vi "Chirp_DFT_V3.vi"(8 "error in (no error)":errorcluster, 11 "ChirpV2 in":refnum<class "ChirpV2.lvclass">) -> (0 "error out":errorcluster, 3 "ChirpV2 out":refnum<class "ChirpV2.lvclass">)   [LabVIEW 2014, in "ChirpV2.lvclass"]
uses:
  ChirpV2.lvclass
  <vilib>/Analysis/2dsp.llb/Real FFT.vi
  <vilib>/Analysis/NI_AALPro.lvlib
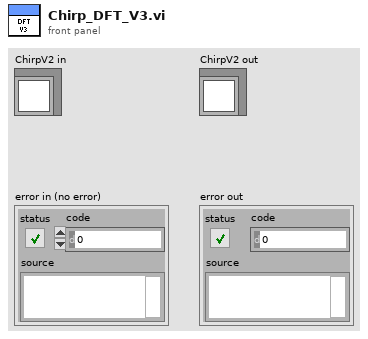
[diagram p1: front panel]
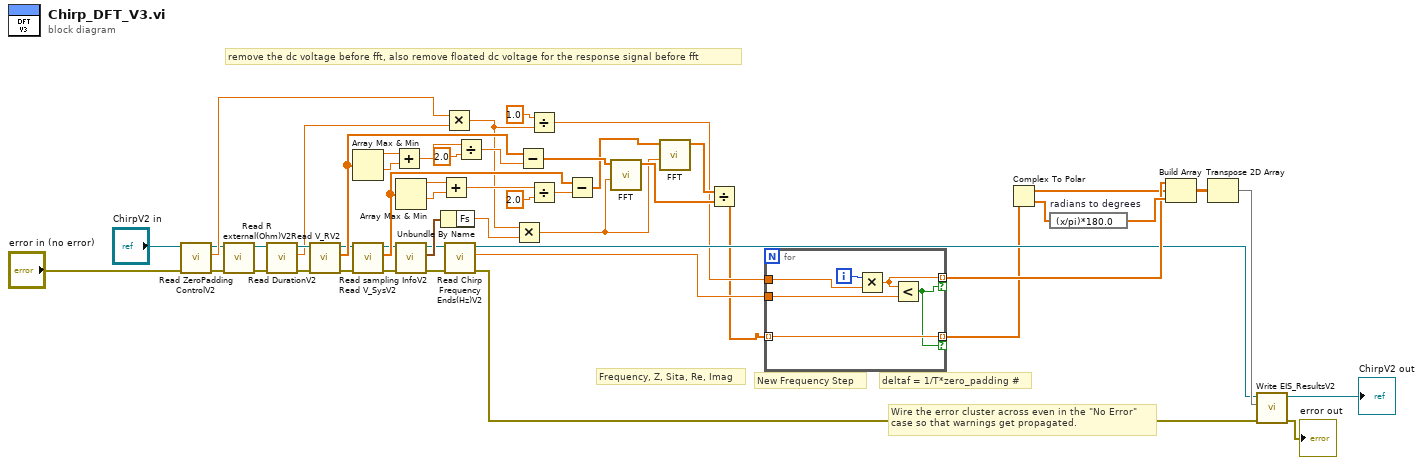
[diagram p0: block diagram]
diagram:
  # "deltaf = 1/T*zero_padding #"
  # "remove the dc voltage before fft, also remove floated dc voltage for the response signal before fft"
  # "Frequency, Z, Sita, Re, Imag"
  # "New Frequency Step"
  # "Wire the error cluster across even in the \"No Error\"\ncase so that warnings get propagated."
  n1 = call-dynamic "Read ZeroPadding ControlV2.vi"("error in (no error)"="error in (no error)", "ChirpV2 in"="ChirpV2 in") -> ("error out"=w49:errorcluster, "ZeroPadding Control"=w50:dbl, "ChirpV2 out"=w48:refnum<class "ChirpV2.lvclass">)  [unwired: 7 in]
  n2 = call-dynamic "Read R external(Ohm)V2.vi"("error in (no error)"=w49, "ChirpV2 in"=w48) -> ("error out"=w19:errorcluster, "ChirpV2 out"=w21:refnum<class "ChirpV2.lvclass">)  [unwired: 7 in, 1 out]
  n3 = call-dynamic "Read DurationV2.vi"("error in (no error)"=w19, "ChirpV2 in"=w21) -> ("error out"=w18:errorcluster, "Duration"=w17:dbl, "ChirpV2 out"=w20:refnum<class "ChirpV2.lvclass">)  [unwired: 7 in]
  n4 = call-dynamic "Read V_RV2.vi"("error in (no error)"=w18, "ChirpV2 in"=w20) -> ("error out"=w41:errorcluster, "V_R"=w42:dbl[], "ChirpV2 out"=w40:refnum<class "ChirpV2.lvclass">)  [unwired: 7 in]
  n5 = Array Max & Min(array=w42) -> (max value=w30:dbl, min value=w31:dbl)  [unwired: 2 out]
  n6 = call-dynamic "Read V_SysV2.vi"("error in (no error)"=w41, "ChirpV2 in"=w40) -> ("error out"=w15:errorcluster, "V_Sys"=w51:dbl[], "ChirpV2 out"=w16:refnum<class "ChirpV2.lvclass">)  [unwired: 7 in]
  n7 = Add(x=w30, y=w31) -> (x+y=w32:dbl)
  n8 = Array Max & Min(array=w51) -> (max value=w37:dbl, min value=w38:dbl)  [unwired: 2 out]
  n9 = call-dynamic "Read sampling InfoV2.vi"("error in (no error)"=w15, "ChirpV2 in"=w16) -> ("error out"=w9:errorcluster, "sampling Info"=w14:cluster{"Fs":dbl}, "ChirpV2 out"=w10:refnum<class "ChirpV2.lvclass">)  [unwired: 7 in]
  n10 = Add(x=w37, y=w38) -> (x+y=w35:dbl)
  n11 = Unbundle By Name(w14) -> ("Fs"=w12:dbl)
  n12 = Multiply(x=w50, y=w17) -> (x*y=w13:dbl)
  n13 = call-dynamic "Read Chirp Frequency Ends(Hz)V2.vi"("error in (no error)"=w9, "ChirpV2 in"=w10) -> ("error out"=w7:errorcluster, "Chirp Frequency Ends(Hz)"=w6:dbl, "ChirpV2 out"=w8:refnum<class "ChirpV2.lvclass">)  [unwired: 7 in]
  n14 = Divide(x=w32, y=2.0) -> (x/y=w34:dbl)
  n15 = Multiply(x=w13, y=w12) -> (x*y=w11:dbl)
  n16 = Subtract(x=w42, y=w34) -> (x-y=w2:dbl[])
  n17 = Divide(x=1.0, y=w13) -> (x/y=w5:dbl)
  n18 = Divide(x=w35, y=2.0) -> (x/y=w39:dbl)
  n19 = Subtract(x=w51, y=w39) -> (x-y=w1:dbl[])
  n20 = call-poly <vilib>:"FFT.vi"("FFT size"=w11, "X"=w2) -> ("FFT {X}"=w22:cdb[])  [unwired: 8 in, 1 out]
  n21 = call-poly <vilib>:"FFT.vi"("FFT size"=w11, "X"=w1) -> ("FFT {X}"=w23:cdb[])  [unwired: 8 in, 1 out]
  n22 = Divide(x=w23, y=w22) -> (x/y=w4:cdb[])
  n23 = for {
    tunnel: w5 -> [w57]
    tunnel: [w55] -> w26 mode=indexing if=w52
    tunnel: w6 -> [w54]
    tunnel: w4 -> [w53] mode=indexing
    tunnel: [w53] -> w3 mode=indexing if=w52
    i -> [w56]
    n24 = Multiply(x=w56, y=w57) -> (x*y=w55:dbl)
    n25 = Less?(x=w55, y=w54) -> (x < y?=w52:bool)
  }
  n26 = Complex To Polar(r * e^(i*theta)=w3) -> (r=w25:dbl[], theta=w28:dbl[])
  n27 = expression code="(x/pi)*180.0" "radians to degrees"(w28) -> (w29:dbl[])
  n28 = Build Array(w26, w25, w29) -> (w24:dbl[][])
  n29 = Transpose 2D Array(2D array=w24) -> (transposed array=w43:dbl[][])
  n30 = call-dynamic "Write EIS_ResultsV2.vi"("error in (no error)"=w7, "EIS_Results"=w43, "ChirpV2 in"=w8) -> ("error out"=→"error out":errorcluster, "ChirpV2 out"=→"ChirpV2 out":refnum<class "ChirpV2.lvclass">)  [unwired: 7 in]
